vi "projekt_pomoc.vi"(5 "String 9":string, 6 "String":string, 7 "String 5":string, 8 "String 2":string, 9 "String 6":string, 10 "String 3":string, 11 "String 7":string, 12 "String 4":string, 13 "String 8":string) -> (17 "x .or. y?":bool, 18 "String 10":string)   [LabVIEW 2023]
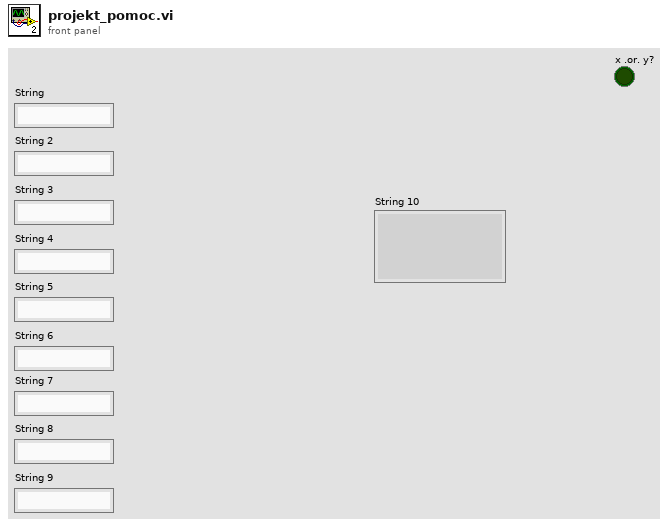
[diagram p1: front panel]
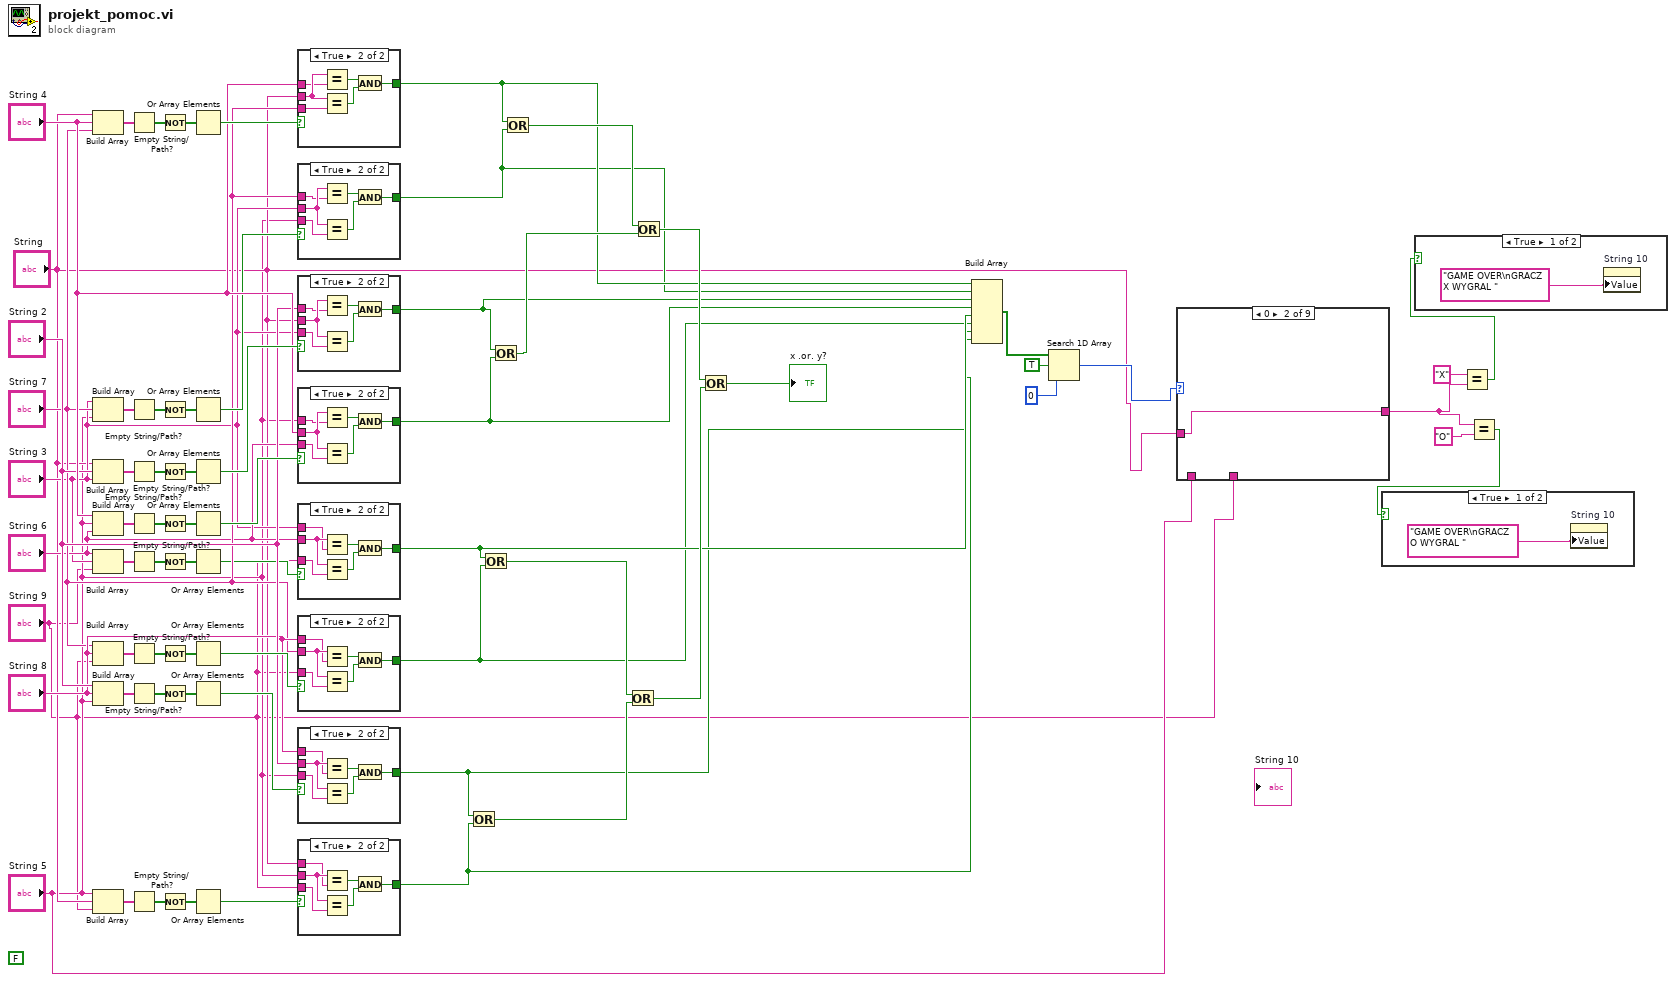
[diagram p0: block diagram]
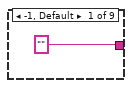
[diagram p4: hidden frame]
diagram:
  (unwired) FALSE
  n1 = Build Array("String", "String 4", "String 7") -> (w53:string[])
  n2 = Build Array("String 3", "String 7", "String 5") -> (w38:string[])
  n3 = Build Array("String", "String 2", "String 3") -> (w65:string[])
  n4 = Build Array("String 4", "String 5", "String 6") -> (w61:string[])
  n5 = Build Array("String 6", "String 3", "String 9") -> (w33:string[])
  n6 = Build Array("String 7", "String 8", "String 9") -> (w57:string[])
  n7 = Build Array("String 2", "String 8", "String 5") -> (w44:string[])
  n8 = Build Array("String 5", "String", "String 9") -> (w48:string[])
  n9 = Empty String/Path?(string/path=w53) -> (empty?=w52:bool[])
  n10 = Empty String/Path?(string/path=w38) -> (empty?=w37:bool[])
  n11 = Empty String/Path?(string/path=w65) -> (empty?=w64:bool[])
  n12 = Empty String/Path?(string/path=w61) -> (empty?=w60:bool[])
  n13 = Empty String/Path?(string/path=w33) -> (empty?=w32:bool[])
  n14 = Empty String/Path?(string/path=w57) -> (empty?=w56:bool[])
  n15 = Empty String/Path?(string/path=w44) -> (empty?=w43:bool[])
  n16 = Empty String/Path?(string/path=w48) -> (empty?=w47:bool[])
  n17 = Not(x=w52) -> (.not. x?=w51:bool[])
  n18 = Not(x=w37) -> (.not. x?=w36:bool[])
  n19 = Not(x=w64) -> (.not. x?=w63:bool[])
  n20 = Not(x=w60) -> (.not. x?=w59:bool[])
  n21 = Not(x=w32) -> (.not. x?=w31:bool[])
  n22 = Not(x=w56) -> (.not. x?=w55:bool[])
  n23 = Not(x=w43) -> (.not. x?=w42:bool[])
  n24 = Not(x=w47) -> (.not. x?=w46:bool[])
  n25 = Or Array Elements(Boolean array=w51) -> (logical OR=w50:bool)
  n26 = Or Array Elements(Boolean array=w36) -> (logical OR=w35:bool)
  n27 = Or Array Elements(Boolean array=w63) -> (logical OR=w62:bool)
  n28 = Or Array Elements(Boolean array=w59) -> (logical OR=w58:bool)
  n29 = Or Array Elements(Boolean array=w31) -> (logical OR=w30:bool)
  n30 = Or Array Elements(Boolean array=w55) -> (logical OR=w54:bool)
  n31 = Or Array Elements(Boolean array=w42) -> (logical OR=w41:bool)
  n32 = Or Array Elements(Boolean array=w46) -> (logical OR=w45:bool)
  n33 = case shown="True" w50 {
    tunnel: "String" -> [_ w71]
    tunnel: "String 4" -> [_ w70]
    tunnel: "String 7" -> [_ w69]
    tunnel: [_ w66] -> w20
    frame False {
    }
    frame True {
      n34 = Equal?(x=w71, y=w70) -> (x = y?=w68:bool)
      n35 = Equal?(x=w71, y=w69) -> (x = y?=w67:bool)
      n36 = And(x=w68, y=w67) -> (x .and. y?=w66:bool)
    }
  }
  n37 = case shown="True" w35 {
    tunnel: "String 3" -> [_ w77]
    tunnel: "String 7" -> [_ w76]
    tunnel: "String 5" -> [_ w75]
    tunnel: [_ w72] -> w19
    frame False {
    }
    frame True {
      n38 = Equal?(x=w77, y=w76) -> (x = y?=w74:bool)
      n39 = Equal?(x=w77, y=w75) -> (x = y?=w73:bool)
      n40 = And(x=w74, y=w73) -> (x .and. y?=w72:bool)
    }
  }
  n41 = case shown="True" w62 {
    tunnel: "String" -> [_ w83]
    tunnel: "String 2" -> [_ w82]
    tunnel: "String 3" -> [_ w81]
    tunnel: [_ w78] -> w18
    frame False {
    }
    frame True {
      n42 = Equal?(x=w83, y=w82) -> (x = y?=w80:bool)
      n43 = Equal?(x=w83, y=w81) -> (x = y?=w79:bool)
      n44 = And(x=w80, y=w79) -> (x .and. y?=w78:bool)
    }
  }
  n45 = case shown="True" w58 {
    tunnel: "String 4" -> [_ w89]
    tunnel: "String 5" -> [_ w88]
    tunnel: "String 6" -> [_ w87]
    tunnel: [_ w84] -> w17
    frame False {
    }
    frame True {
      n46 = Equal?(x=w89, y=w88) -> (x = y?=w86:bool)
      n47 = Equal?(x=w89, y=w87) -> (x = y?=w85:bool)
      n48 = And(x=w86, y=w85) -> (x .and. y?=w84:bool)
    }
  }
  n49 = case shown="True" w30 {
    tunnel: "String 6" -> [_ w95]
    tunnel: "String 3" -> [_ w94]
    tunnel: "String 9" -> [_ w93]
    tunnel: [_ w90] -> w16
    frame False {
    }
    frame True {
      n50 = Equal?(x=w95, y=w94) -> (x = y?=w92:bool)
      n51 = Equal?(x=w95, y=w93) -> (x = y?=w91:bool)
      n52 = And(x=w92, y=w91) -> (x .and. y?=w90:bool)
    }
  }
  n53 = case shown="True" w54 {
    tunnel: "String 7" -> [_ w101]
    tunnel: "String 8" -> [_ w100]
    tunnel: "String 9" -> [_ w99]
    tunnel: [_ w96] -> w15
    frame False {
    }
    frame True {
      n54 = Equal?(x=w101, y=w100) -> (x = y?=w98:bool)
      n55 = Equal?(x=w101, y=w99) -> (x = y?=w97:bool)
      n56 = And(x=w98, y=w97) -> (x .and. y?=w96:bool)
    }
  }
  n57 = case shown="True" w41 {
    tunnel: "String 2" -> [_ w107]
    tunnel: "String 8" -> [_ w106]
    tunnel: "String 5" -> [_ w105]
    tunnel: [_ w102] -> w14
    frame False {
    }
    frame True {
      n58 = Equal?(x=w107, y=w106) -> (x = y?=w104:bool)
      n59 = Equal?(x=w107, y=w105) -> (x = y?=w103:bool)
      n60 = And(x=w104, y=w103) -> (x .and. y?=w102:bool)
    }
  }
  n61 = case shown="True" w45 {
    tunnel: "String 5" -> [_ w113]
    tunnel: "String" -> [_ w112]
    tunnel: "String 9" -> [_ w111]
    tunnel: [_ w108] -> w13
    frame False {
    }
    frame True {
      n62 = Equal?(x=w113, y=w112) -> (x = y?=w110:bool)
      n63 = Equal?(x=w113, y=w111) -> (x = y?=w109:bool)
      n64 = And(x=w110, y=w109) -> (x .and. y?=w108:bool)
    }
  }
  n65 = Or(x=w14, y=w13) -> (x .or. y?=w24:bool)
  n66 = Or(x=w16, y=w15) -> (x .or. y?=w25:bool)
  n67 = Or(x=w18, y=w17) -> (x .or. y?=w26:bool)
  n68 = Or(x=w20, y=w19) -> (x .or. y?=w27:bool)
  n69 = Or(x=w25, y=w24) -> (x .or. y?=w22:bool)
  n70 = Or(x=w27, y=w26) -> (x .or. y?=w23:bool)
  n71 = Or(x=w23, y=w22) -> (x .or. y?=→"x .or. y?":bool)
  n72 = Build Array(w20, w19, w18, w17, w16, w15, w14, w13) -> (w12:bool[])
  n73 = Search 1D Array(1D array=w12, element=TRUE, start index (0)=0) -> (index of element=w9:i32)
  n74 = case shown="0" w9 {
    tunnel: "String" -> [_ w115 _ w117 _ _ _ _ w122]
    tunnel: "String 5" -> [_ _ w116 _ w118 _ _ w121 _]
    tunnel: "String 9" -> [_ _ _ _ _ w119 w120 _ _]
    tunnel: ["" w115 w116 w117 w118 w119 w120 w121 w122] -> w1
    frame -1, Default {
    }
    frame 0 {
    }
    frame 1 {
    }
    frame 2 {
    }
    frame 3 {
    }
    frame 4 {
    }
    frame 5 {
    }
    frame 6 {
    }
    frame 7 {
    }
  }
  n75 = Equal?(x="X", y=w1) -> (x = y?=w3:bool)
  n76 = case shown="True" w3 {
    frame True {
      n77 = property on="String 10" class="Str"("Value"="GAME OVER\nGRACZ X WYGRAL ") -> ()  [unwired: 2 in, 2 out]
    }
    frame False {
    }
  }
  n78 = Equal?(x=w1, y="O") -> (x = y?=w2:bool)
  n79 = case shown="True" w2 {
    frame True {
      n80 = property on="String 10" class="Str"("Value"="GAME OVER\nGRACZ O WYGRAL ") -> ()  [unwired: 2 in, 2 out]
    }
    frame False {
    }
  }
